vi "new BombedWall.vi"(8 "error in (no error)":errorcluster) -> (0 "error out":errorcluster, 3 "BombedWall* out":T1)   [LabVIEW 2016, in "BombedWall.lvclass"]
uses:
  BombedWall.lvclass
  BombedWall Reference.ctl
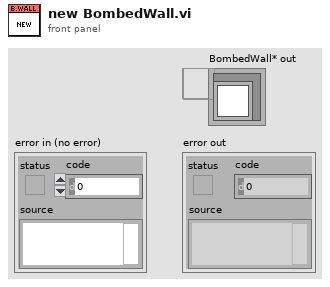
[diagram p1: front panel]
types:
  T1 = typedef "BombedWall.lvclass/BombedWall Reference.ctl" = refnum<data-value>
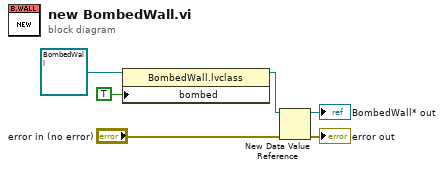
[diagram p0: block diagram]
diagram:
  n1 = property class="BombedWall.lvclass"(reference=refnum<class "BombedWall.lvclass"> refnum ("BombedWall in"), "bombed"=TRUE) -> (reference out=w2:refnum<class "BombedWall.lvclass">)  [unwired: 1 in, 1 out]
  n2 = New Data Value Reference(data value=w2, error in="error in (no error)") -> (data value reference=→"BombedWall* out":refnum<data-value>, error out=→"error out":errorcluster)
